vi "SetAttributeViInt32.vi"(7 "AttributeValue":i32 format="%.0g", 8 "error in (no error)":errorcluster {"code" format="%.0x"}, 9 "AttributeID":u32(ring)=1250001 items=["AMPLITUDE_UNITS"=1250001, "ANALOGDEMODULATOR_FM_DE_EMPHASIS"=1150560, "ANALOGDEMODULATOR_TYPE"=1150556, "CALIBRATION_AUTO_ALERT_MODE"=1150674, "CALIBRATION_AUTO_ENABLED"=1150675, "DETECTOR_TYPE"=1250004, "DISPLAY_NORMALIZED_POSITION"=1150188, "DISPLAY_OPERATION_PRIORITY"=1150742, "DISPLAY_THEME"=1150155, "DISPLAY_VIEW"=1150743, "DISPLAY_WINDOW"=1150181, "EXTERNAL_MIXER_HARMONIC"=1250907, "EXTERNAL_MIXER_NUMBER_OF_PORTS"=1250908, "EXTERNAL_TRIGGER_SLOPE"=1250402, "FORMAT"=1150876, "FREQUENCY_SYNTHESIS"=1150543, "INPUT_AMPLITUDE_REFERENCE"=1150562, "INPUT_IF_FFT_IF_GAIN_STATE"=1150565, "INPUT_IF_SWEPT_IF_GAIN_STATE"=1150568, "INPUT_PORT"=1150563, "INPUT_RF_CORRECTION_ANTENNA_UNIT"=1150736, "INPUT_RF_CORRECTION_FREQUENCY_INTERPOLATION"=1150575, "INPUT_RF_CORRECTIONS_IMPEDANCE"=1150739, "INPUT_RF_COUPLING"=1150571, "INPUT_TYPE"=1150774, "OUTPUT_TYPE"=1150921, "REFERENCE_TYPE"=1150852, "SCALE_TYPE"=1150811], 10 "RepCapIdentifier":string, 11 "instrument handle":refnum<k15>) -> (0 "error out":errorcluster {"code" format="%.0x"}, 3 "instrument handle out":refnum<k15>)   [LabVIEW 2009, in "Keysight XSAn.lvlib"]
doc: "Sets an Int32 attribute from the instrument driver.\nThe following Attributes are supported:\n\nAMPLITUDE_UNITS\nANALOGDEMODULATOR_FM_DE_EMPHASIS\nANALOGDEMODULATOR_TYPE\nCALIBRATION_AUTO_ALERT_MODE\nCALIBRATION_AUTO_ENABLED\nDETECTOR_TYPE\nDISPLAY_NORMALIZED_POSITION\nDISPLAY_OPERATION_PRIORITY\nDISPLAY_THEME\nDISPLAY_VIEW\nDISPLAY_WINDOW\nEXTERNAL_MIXER_HARMONIC\nEXTERNAL_MIXER_NUMBER_OF_PORTS\nEXTERNAL_TRIGGER_SLOPE\nFORMAT\nFREQUENCY_SYNTHESIS\nINPUT_AMPLITUDE_REFERENCE\nINPUT_IF_FFT_IF_GAIN_STATE\nINPUT_IF_SWEPT_IF_GAIN_STATE\nINPUT_PORT\nINPUT_RF_CORRECTION_ANTENNA_UNIT\nINPUT_RF_CORRECTION_FREQUENCY_INTERPOLATION\nINPUT_RF_CORRECTIONS_IMPEDANCE\nINPUT_RF_COUPLING\nINPUT_TYPE\nOUTPUT_TYPE\nREFERENCE_TYPE \nSCALE_TYPE"
uses:
  <instrlib>/Keysight XSAn/Keysight XSAn.lvlib
  AgXSAn.dll
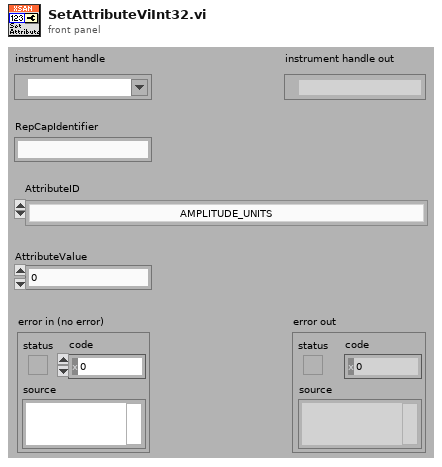
[diagram p1: front panel]
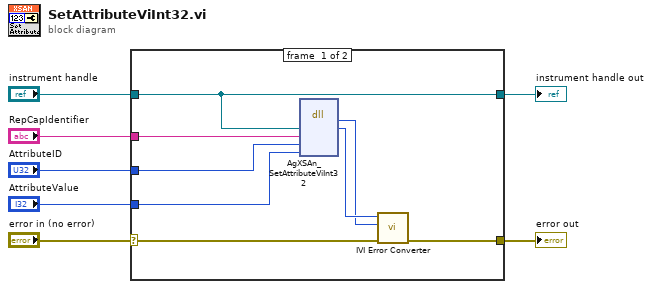
[diagram p0: block diagram]
diagram:
  n1 = case shown="No Error" "error in (no error)" {
    selector: "error in (no error)" -> [w13 w17]
    tunnel: [w12 w17] -> w7
    tunnel: "instrument handle" -> [w8 w16]
    tunnel: "RepCapIdentifier" -> [w11 _]
    tunnel: "AttributeID" -> [w10 _]
    tunnel: "AttributeValue" -> [w9 _]
    tunnel: [w8 w16] -> w1
    frame #0 {
      n2 = dll-call lib="AgXSAn**.dll" fn="AgXSAn_SetAttributeViInt32"("Vi"=w8, "RepCapIdentifier"=w11, "AttributeID"=w10, "AttributeValue"=w9) -> ("return type"=w14:i32, "Vi"=w15:u32)  [unwired: 6 in, 2 out]
      n3 = call <instrlib>:"IVI Error Converter.vi"("error in (no error)"=w13, "IVI error code (0)"=w14, "instrument handle"=w15) -> ("error out"=w12:errorcluster)  [unwired: 7 in, 1 out]
    }
    frame #1 {
    }
  }
  "error out" <- w7
  "instrument handle out" <- w1
